vi "close.vi"(8 "error in (no error)":errorcluster, 11 "ADODB._Connection In":refnum<k7>) -> (0 "error out":errorcluster)   [LabVIEW 2016, in "database.lvlib"]
uses:
  database.lvlib
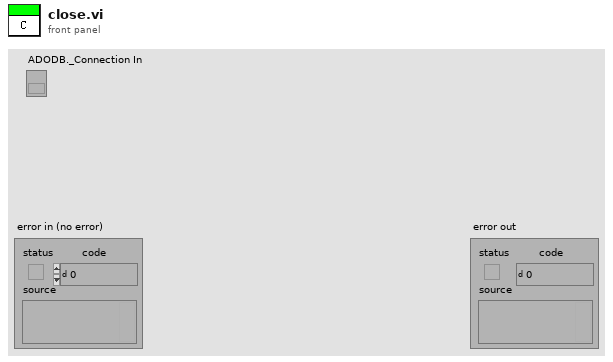
[diagram p1: front panel]
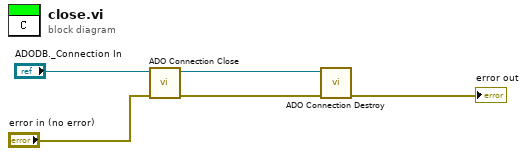
[diagram p0: block diagram]
diagram:
  n1 = call <userlib>:"ADO Connection Close.vi"("error in (no error)"="error in (no error)", "ADODB._Connection In"="ADODB._Connection In") -> ("error out"=w4:errorcluster, "ADODB._Connection Out"=w5:refnum<k7>)  [unwired: 8 in]
  n2 = call <userlib>:"ADO Connection Destroy.vi"("error in (no error)"=w4, "ADODB._Connection In"=w5) -> ("error out"=→"error out":errorcluster)  [unwired: 9 in]
